vi "Material.Decode Palette Array.vi"(11 "Palettes":refnum<class "Material-Palette.lvclass">) -> (2 "palette":T1={"0"="0", "5"="0", "10"="0", "15"="0", "20"="0", "25"="0", "30"="0", "35"="0", "40"="0", "50"="0", "60"="0", "70"="0", "80"="0", "90"="0", "95"="0", "98"="0", "99"="0", "100"="0"})   [LabVIEW 2021, in "TSC Material Theme.lvlib" / "Material-Palette.lvclass"]
doc: "Convert the json represenation of the palette colors into array of class palettes.\n\n<b>Code Developed By:</b> +\nDaniel Coons +\nTechnology Service Corporation +\nwww.tsc.com/atcs"
uses:
  Material-Palette.lvclass
  Material-Palette.lvclass/Material-Palette.ctl
  TSC Material Theme/material json palette--cluster.ctl
  TSC Material Theme/TSC Material Theme.lvlib
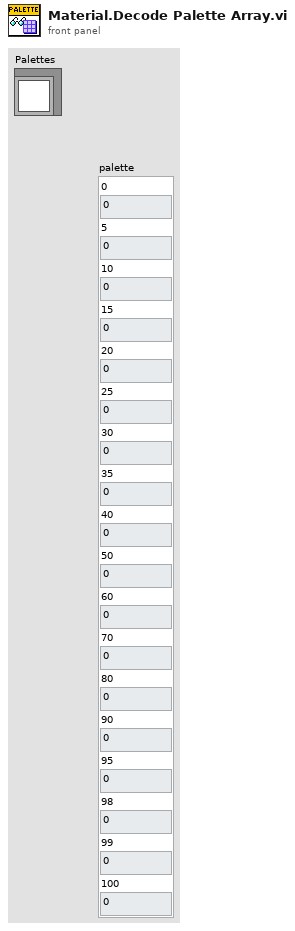
[diagram p1: front panel]
types:
  T1 = typedef "TSC Material Theme.lvlib/material json palette--cluster.ctl" = cluster{"0":string, "5":string, "10":string, "15":string, "20":string, "25":string, "30":string, "35":string, "40":string, "50":string, "60":string, "70":string, "80":string, "90":string, "95":string, "98":string, "99":string, "100":string}
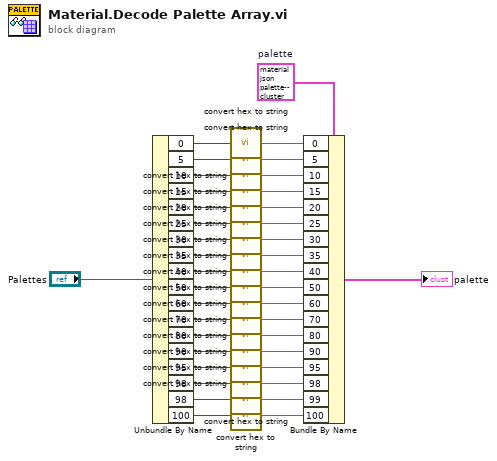
[diagram p0: block diagram]
diagram:
  w39 = T1 {"0"="0", "5"="0", "10"="0", "15"="0", "20"="0", "25"="0", "30"="0", "35"="0", "40"="0", "50"="0", "60"="0", "70"="0", "80"="0", "90"="0", "95"="0", "98"="0", "99"="0", "100"="0"}  # palette
  n1 = Unbundle By Name("Palettes") -> ("0"=w36:u32, "5"=w34:u32, "10"=w31:u32, "15"=w30:u32, "20"=w27:u32, "25"=w26:u32, "30"=w24:u32, "35"=w21:u32, "40"=w20:u32, "50"=w18:u32, "60"=w16:u32, "70"=w14:u32, "80"=w12:u32, "90"=w11:u32, "95"=w10:u32, "98"=w9:u32, "98"=w8:u32, "100"=w7:u32)
  n2 = call "convert hex to string.vi"("hex"=w36) -> ("string"=w35:string)
  n3 = call "convert hex to string.vi"("hex"=w34) -> ("string"=w33:string)
  n4 = call "convert hex to string.vi"("hex"=w31) -> ("string"=w32:string)
  n5 = call "convert hex to string.vi"("hex"=w30) -> ("string"=w29:string)
  n6 = call "convert hex to string.vi"("hex"=w27) -> ("string"=w28:string)
  n7 = call "convert hex to string.vi"("hex"=w26) -> ("string"=w25:string)
  n8 = call "convert hex to string.vi"("hex"=w24) -> ("string"=w23:string)
  n9 = call "convert hex to string.vi"("hex"=w21) -> ("string"=w22:string)
  n10 = call "convert hex to string.vi"("hex"=w20) -> ("string"=w19:string)
  n11 = call "convert hex to string.vi"("hex"=w18) -> ("string"=w17:string)
  n12 = call "convert hex to string.vi"("hex"=w16) -> ("string"=w15:string)
  n13 = call "convert hex to string.vi"("hex"=w14) -> ("string"=w13:string)
  n14 = call "convert hex to string.vi"("hex"=w12) -> ("string"=w1:string)
  n15 = call "convert hex to string.vi"("hex"=w11) -> ("string"=w2:string)
  n16 = call "convert hex to string.vi"("hex"=w10) -> ("string"=w3:string)
  n17 = call "convert hex to string.vi"("hex"=w9) -> ("string"=w4:string)
  n18 = call "convert hex to string.vi"("hex"=w8) -> ("string"=w5:string)
  n19 = call "convert hex to string.vi"("hex"=w7) -> ("string"=w6:string)
  n20 = Bundle By Name(cluster=w39, "0"=w35, "5"=w33, "10"=w32, "15"=w29, "20"=w28, "25"=w25, "30"=w23, "35"=w22, "40"=w19, "50"=w17, "60"=w15, "70"=w13, "80"=w1, "90"=w2, "95"=w3, "98"=w4, "99"=w5, "100"=w6) -> (→"palette":T1)
